vi "PNA fetch s-parameters.vi"() -> ()   [LabVIEW 2020]
uses:
  Instruments/Vector Network Analyzer/Controls/Sparameter cluster.ctl
  Instruments/Vector Network Analyzer/Vector Network Analyzer.lvclass
  <instrlib>/Agilent PNA Series/Agilent PNA Series.lvlib
panel:
  in  "x":dbl
  in  "VISA resource name":refnum<visa-resource-name>
  in  "length":i32
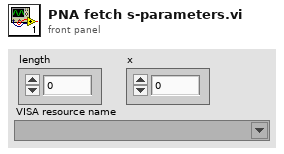
[diagram p1: front panel]
types:
  T1 = typedef "Vector Network Analyzer.lvclass/Sparameter cluster.ctl" = cluster{"Frequency":dbl, "S Parameters":cdb[]}
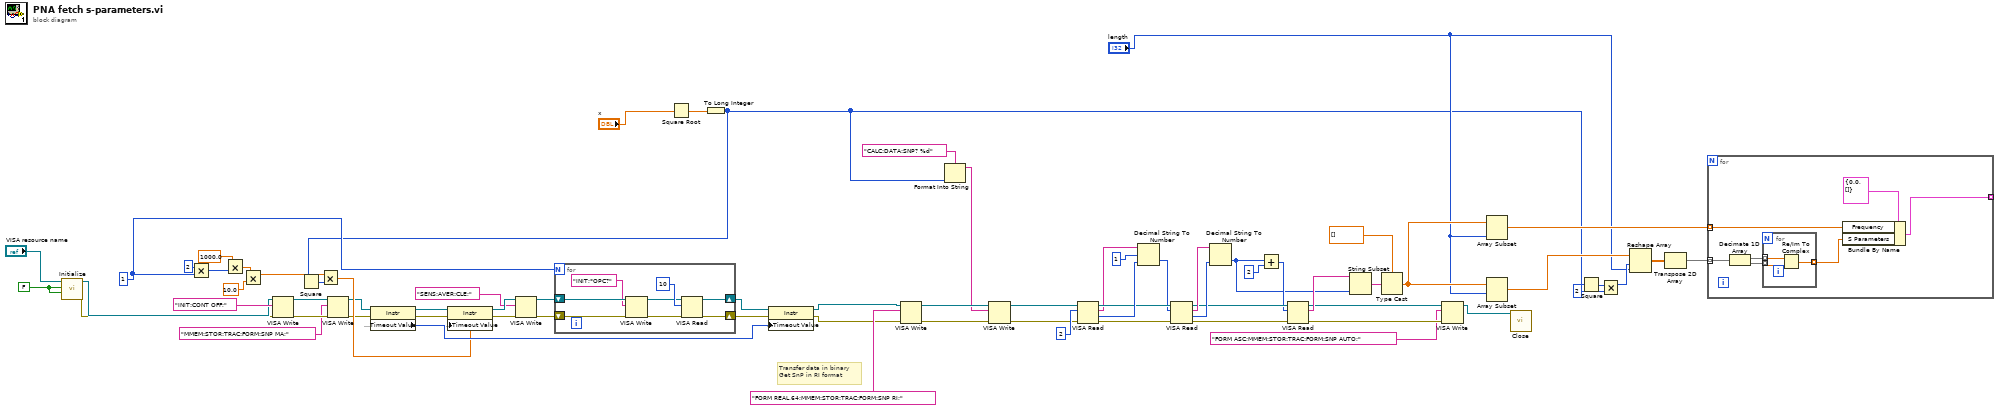
[diagram p0: block diagram]
diagram:
  w8 = FALSE ("ID Query (T: Check)")
  w16 = 1 ("f")
  # "Transfer data in binary\nGet SnP in RI format"
  n1 = call <instrlib>:"Initialize.vi"("Reset (T: Reset)"=w8, "ID Query (T: Check)"=w8, "Instrument Resource Name"="VISA resource name") -> ("error out"=w5:errorcluster, "dup VISA session"=w7:refnum<visa-resource-name>)  [unwired: 7 in]
  n2 = Multiply(x=2 ("x 2"), y=w16) -> (x*y=w30:i32)
  n3 = Multiply(x=1000.0, y=w30) -> (x*y=w29:dbl)
  n4 = Multiply(x=w29, y=10.0) -> (x*y=w25:dbl)
  n5 = VISA Write(VISA resource name=w7, write buffer="INIT:CONT OFF;", error in (no error)=w5) -> (VISA resource name out=w11:refnum<visa-resource-name>, error out=w10:errorcluster)  [unwired: 1 out]
  n6 = VISA Write(VISA resource name=w11, write buffer="MMEM:STOR:TRAC:FORM:SNP MA;", error in (no error)=w10) -> (VISA resource name out=w12:refnum<visa-resource-name>, error out=w13:errorcluster)  [unwired: 1 out]
  n7 = property class="Instr"(reference=w12, error in=w13) -> (reference out=w32:refnum<visa-resource-name>, error out=w31:errorcluster, "General Settings:Timeout Value"=w22:u32)
  n8 = Square Root(x="x") -> (sqrt(x)=w36:dbl)
  n9 = To Long Integer(number=w36) -> (32bit integer=w2:i32)
  n10 = Square(x=w2) -> (x^2=w14:i32)
  n11 = Multiply(x=w25, y=w14) -> (x*y=w15:dbl)
  n12 = property class="Instr"(reference=w32, error in=w31, "General Settings:Timeout Value"=w15) -> (reference out=w27:refnum<visa-resource-name>, error out=w26:errorcluster)
  n13 = VISA Write(VISA resource name=w27, write buffer="SENS:AVER:CLE;", error in (no error)=w26) -> (VISA resource name out=w19:refnum<visa-resource-name>, error out=w20:errorcluster)  [unwired: 1 out]
  n14 = for {
    N: w16 -> [_]
    shift-right: [w78] -> w21
    shift-left: w20 -> [w76]
    shift-right: [w79] -> w23
    shift-left: w19 -> [w75]
    n15 = VISA Write(VISA resource name=w75, write buffer="INIT;*OPC?", error in (no error)=w76) -> (VISA resource name out=w74:refnum<visa-resource-name>, error out=w73:errorcluster)  [unwired: 1 out]
    n16 = VISA Read(VISA resource name=w74, byte count=u32 10, error in (no error)=w73) -> (VISA resource name out=w79:refnum<visa-resource-name>, error out=w78:errorcluster)  [unwired: 2 out]
  }
  n17 = property class="Instr"(reference=w23, error in=w21, "General Settings:Timeout Value"=w22) -> (reference out=w3:refnum<visa-resource-name>, error out=w4:errorcluster)
  n18 = VISA Write(VISA resource name=w3, write buffer="FORM REAL,64;MMEM:STOR:TRAC:FORM:SNP RI;", error in (no error)=w4) -> (VISA resource name out=w69:refnum<visa-resource-name>, error out=w70:errorcluster)  [unwired: 1 out]
  n19 = Format Into String(format string="CALC:DATA:SNP? %d", w2) -> (resulting string=w67:string)  [unwired: 2 in, 1 out]
  n20 = VISA Write(VISA resource name=w69, write buffer=w67, error in (no error)=w70) -> (VISA resource name out=w54:refnum<visa-resource-name>, error out=w55:errorcluster)  [unwired: 1 out]
  n21 = VISA Read(VISA resource name=w54, byte count=u32 2, error in (no error)=w55) -> (VISA resource name out=w63:refnum<visa-resource-name>, read buffer=w46:string, return count=w65:u32, error out=w64:errorcluster)
  n22 = Decimal String To Number(string=w46, offset=1 ("offset (0)"), default (0L)=w65) -> (number=w62:u32)  [unwired: 1 out]
  n23 = VISA Read(VISA resource name=w63, byte count=w62, error in (no error)=w64) -> (VISA resource name out=w58:refnum<visa-resource-name>, read buffer=w60:string, return count=w59:u32, error out=w56:errorcluster)
  n24 = Decimal String To Number(string=w60, default (0L)=w59) -> (number=w49:u32)  [unwired: 1 in, 1 out]
  n25 = Add(x=w49, y=u32 2) -> (x+y=w57:u32)
  n26 = VISA Read(VISA resource name=w58, byte count=w57, error in (no error)=w56) -> (VISA resource name out=w51:refnum<visa-resource-name>, read buffer=w53:string, error out=w52:errorcluster)  [unwired: 1 out]
  n27 = String Subset(string=w53, length (rest)=w49) -> (substring=w44:string)  [unwired: 1 in]
  n28 = Type Cast(type=dbl[] [], x=w44) -> (*(type *) &x=w43:dbl[])
  n29 = VISA Write(VISA resource name=w51, write buffer="FORM ASC;MMEM:STOR:TRAC:FORM:SNP AUTO;", error in (no error)=w52) -> (VISA resource name out=w33:refnum<visa-resource-name>)  [unwired: 2 out]
  n30 = Array Subset(array=w43, length="length") -> (w48:dbl[])  [unwired: 1 in]
  n31 = Array Subset(array=w43, index="length") -> (w39:dbl[])  [unwired: 1 in]
  n32 = call <instrlib>:"Close.vi"("VISA Resource Name"=w33) -> ()  [unwired: 10 in, 1 out]
  n33 = Square(x=w2) -> (x^2=w42:i32)
  n34 = Multiply(x=w42, y=2) -> (x*y=w38:i32)
  n35 = Reshape Array(w39, w38, "length") -> (w40:dbl[][])
  n36 = Transpose 2D Array(2D array=w40) -> (transposed array=w41:dbl[][])
  n37 = for {
    tunnel: w48 -> [w84] mode=indexing
    tunnel: w41 -> [w83] mode=indexing
    tunnel: [w85] -> _ mode=indexing
    n38 = Decimate 1D Array(w83) -> (w82:dbl[], w81:dbl[])
    n39 = for {
      tunnel: w82 -> [w89] mode=indexing
      tunnel: w81 -> [w88] mode=indexing
      tunnel: [w87] -> w80 mode=indexing
      n40 = Re/Im To Complex(1:w88, 2:w89) -> (0:w87:cdb)
    }
    n41 = Bundle By Name(cluster=T1 {"Frequency"=0.0, "S Parameters"=[]} ("S Parameters"), "Frequency"=w84, "S Parameters"=w80) -> (w85:T1)
  }
